vi "Generate daily folder path.vi"(8 "error in (no error)":errorcluster) -> (0 "error out":errorcluster)   [LabVIEW 2020]
uses:
  Global Variables/General Globals.vi
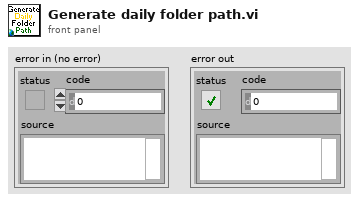
[diagram p1: front panel]
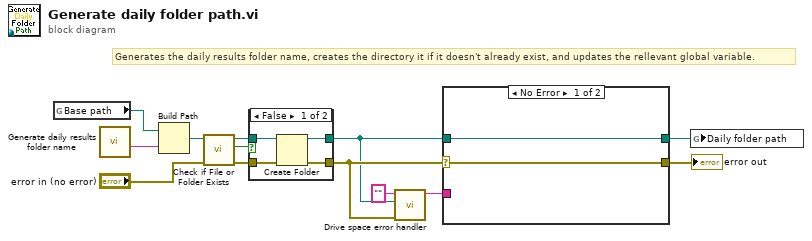
[diagram p0: block diagram]
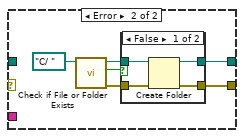
[diagram p2: hidden frame]
diagram:
  # "Generates the daily results folder name, creates the directory it if it doesn't already exist, and updates the rellevant global variable."
  n1 = global read "General Globals.vi" "Base path"() -> (w9:path)
  n2 = call "Generate daily results folder name.vi"() -> ("Generated daily folder name"=w7:string)  [unwired: 11 in]
  n3 = Build Path(base path=w9, name or relative path=w7) -> (appended path=w10:path)
  n4 = call <vilib>:"Check if File or Folder Exists.vi"("error in (no error)"="error in (no error)", "path"=w10) -> ("error out"=w13:errorcluster, "file or folder exists?"=w11:bool, "dup path"=w12:path)  [unwired: 7 in]
  n5 = case shown="False" w11 {
    tunnel: [w16 w19] -> w1
    tunnel: w12 -> [w17 w19]
    tunnel: w13 -> [w15 w18]
    tunnel: [w14 w18] -> w5
    frame False {
      n6 = Create Folder(path (use dialog)=w17, error in=w15) -> (created path=w16:path, error out=w14:errorcluster)  [unwired: 1 in, 1 out]
    }
    frame True {
    }
  }
  n7 = call "Drive space error handler.vi"("error in (no error)"=w5, "Saves folder path"=w1, "String in"="") -> ("String out"=w4:string)  [unwired: 7 in, 1 out]
  n8 = case shown="No Error" w5 {
    selector: w5 -> [w20 _]
    tunnel: w4 -> [_ _]
    tunnel: [w20 w23] -> w3
    tunnel: [w21 w22] -> w2
    tunnel: w1 -> [w21 _]
    frame No Error {
    }
    frame Error {
      n9 = call <vilib>:"Check if File or Folder Exists.vi"("path"=path "C:/ " ("Base path")) -> ("error out"=w25:errorcluster, "file or folder exists?"=w27:bool, "dup path"=w26:path)  [unwired: 8 in]
      n10 = case shown="False" w27 {
        tunnel: [w30 w33] -> w22
        tunnel: w26 -> [w31 w33]
        tunnel: w25 -> [w29 w32]
        tunnel: [w28 w32] -> w23
        frame False {
          n11 = Create Folder(path (use dialog)=w31, error in=w29) -> (created path=w30:path, error out=w28:errorcluster)  [unwired: 1 in, 1 out]
        }
        frame True {
        }
      }
    }
  }
  "error out" <- w3
  n12 = global write "General Globals.vi" "Daily folder path"(w2) -> ()
